vi "FPGA_FSR.vi"() -> ()   [LabVIEW 2019]
uses:
  <vilib>/rvi/Emulation/niFpgaGetClockAttributes.vi
  <vilib>/rvi/Emulation/niFpgaSctlEmulationGetInTimedLoop.vi
  <vilib>/rvi/Emulation/niFpgaEmulationReportErrorSimple.vi
  <vilib>/rvi/eio/common/nirviEmuTemplateMethod_errors.vi
  <vilib>/rvi/Emulation/niFpgaCriticalErrorInLSC.vi
  <vilib>/eio/EIONode/EIONode.xnode
panel:
  out "ConnectorA/AI3":u16
  out "ConnectorA/AI2":u16
  out "ConnectorA/AI1":u16
  out "ConnectorA/AI0":u16
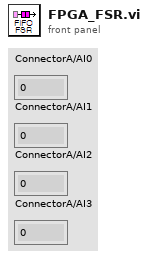
[diagram p1: front panel]
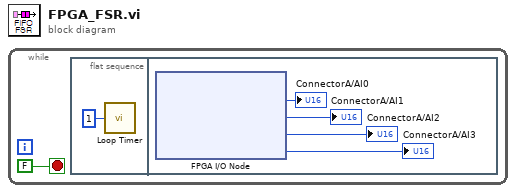
[diagram p0: block diagram]
diagram:
  n1 = while {
    stop <- FALSE stop-if-true
    n2 = flat-sequence {
      frame #0 {
        n3 = call "Loop Timer"("Count(mSec)"=u32 1) -> ()  [unwired: 1 out]
      }
      frame #1 {
        n4 = xnode "FPGA I/O Node"() -> ("ConnectorA/AI0"=→"ConnectorA/AI0":u16, "ConnectorA/AI1"=→"ConnectorA/AI1":u16, "ConnectorA/AI2"=→"ConnectorA/AI2":u16, "ConnectorA/AI3"=→"ConnectorA/AI3":u16)  [unwired: 4 in, 4 out]
      }
    }
  }
